vi "Acquire and Playback Data and Video LV2009.vi"() -> ()   [LabVIEW 2017]
uses:
  <vilib>/userdefined/High Color/IMAQdx.ctl
  <vilib>/DAQmx/read.llb/DAQmx Read (Analog Wfm 1Chan NSamp).vi
  <vilib>/DAQmx/create/channels.llb/DAQmx Create Channel (AI-Acceleration-Accelerometer).vi
  <vilib>/DAQmx/configure/timing.llb/DAQmx Timing (Sample Clock).vi
  <vilib>/DAQmx/miscellaneous.llb/DAQmx Fill In Error Info.vi
  <vilib>/vision/driver/NI_Vision_Acquisition_Software.lvlib
  <resource>/objmgr/daqmx.rc
panel:
  in  "Physical Channels":tag
  in  "AVI Path":path
  in  "Sampling Rate":dbl=1652.0
  in  "Stop Playback":bool
  in  "Tab Control":enum32{"Live Recording", "Playback"}(tab)
  out "Waveform Chart":waveform(dbl)(graph)={"t0"=timestamp(3330377079.0471377 s since 1904-01-01), "dt"=0.0005859375, "Y"=[0.0017552654709999996, 0.0017790570699999996, 0.0017997984639999997, 0.0018540921129999997, 0.0018882544089999997, 0.002001111994, 0.0019730501079999996, 0.0020255136339999997, 0.0021456917109999997, 0.0021944949909999995], "attributes"=variant("NI_ChannelName"=variant(string "cDAQ2Mod4/ai1"), "NI_UnitDescription"=variant(string "g"), "NI_dBReference"=variant(dbl 1.0))}
  out "Acquisition Video":T1(plugin-control)
  out "Waveform Chart 2":waveform(dbl)(graph)
  out "Playback Video":T1(plugin-control)
  out "Movie Progression":dbl(slide) max=500.0 scale=-1.0..335.0
  in  "Stop Acquisition":bool
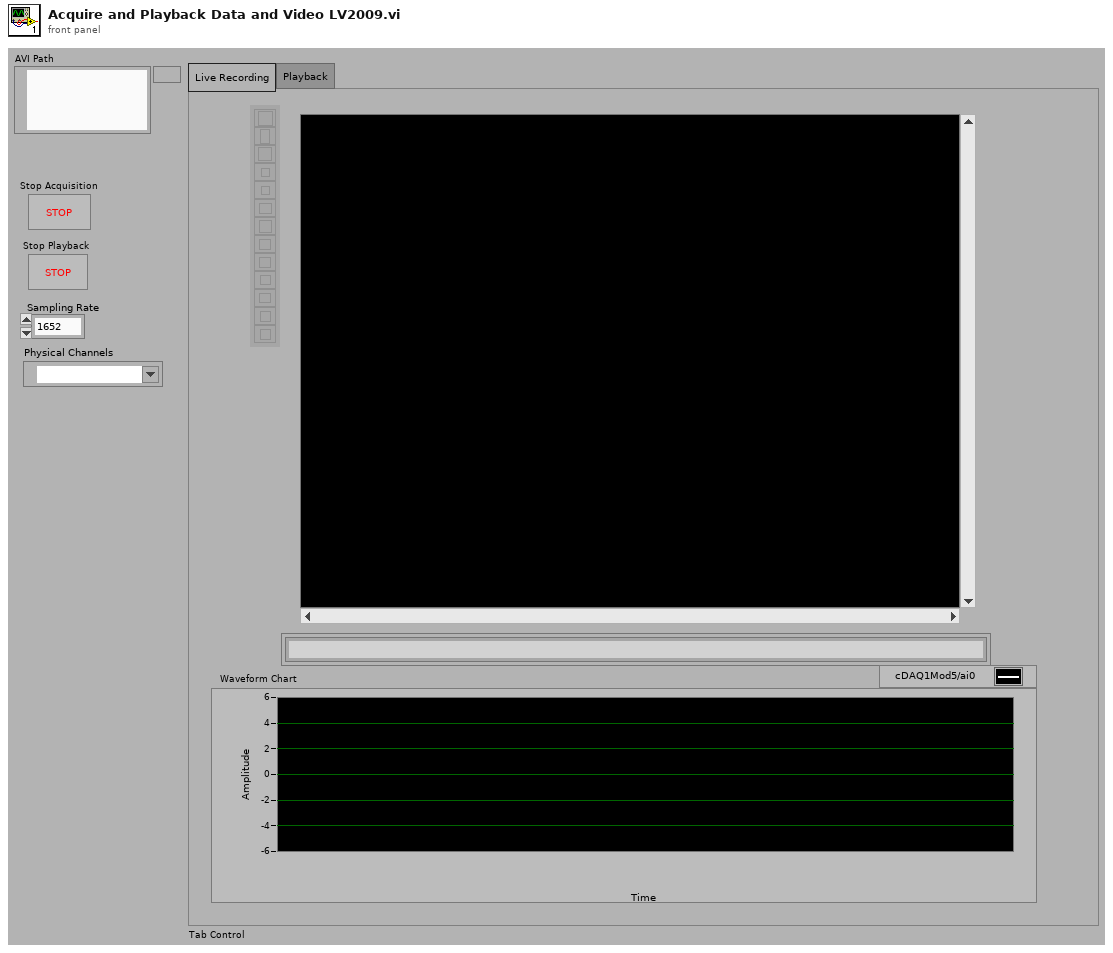
[diagram p1: front panel]
types:
  T1 = typedef "IMAQ Image.ctl" = refnum<image>
  T2 = typedef "IMAQdx.ctl" = refnum<k21>
  T3 = typedef "Image Type" = u32
  T4 = typedef "AviRefnum.ctl" = refnum<k1>
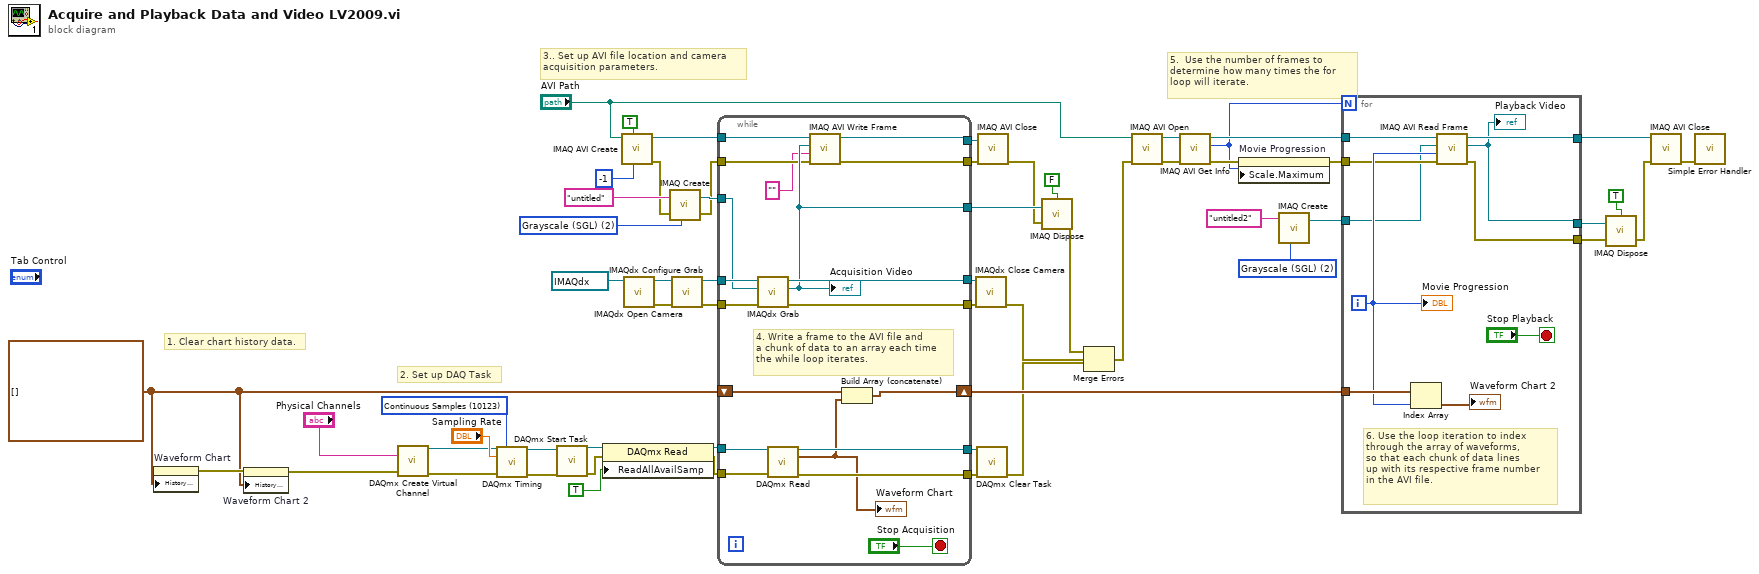
[diagram p0: block diagram]
diagram:
  w2 = waveform(dbl)[] [] ("History Data")
  w29 = T3 2 items=["Grayscale (U8)", "Grayscale (I16)", "Grayscale (SGL)", "Complex (CSG)", "RGB (U32)", "HSL (U32)", "RGB (U64)", "Grayscale (U16)"] ("Image Type")
  w35 = T3 2 items=["Grayscale (U8)", "Grayscale (I16)", "Grayscale (SGL)", "Complex (CSG)", "RGB (U32)", "HSL (U32)", "RGB (U64)", "Grayscale (U16)"] ("Image Type")
  w50 = 10123 items=["Finite Samples"=10178, "Continuous Samples"=10123, "Hardware Timed Single Point"=12522] ("sample mode")
  # "5.  Use the number of frames to \ndetermine how many times the for \nloop will iterate."
  # "3.. Set up AVI file location and camera \nacquisition parameters."
  # "2. Set up DAQ Task"
  # "1. Clear chart history data."
  n1 = property on="Waveform Chart" class="WFChart (strict)"("History Data"=w2) -> (error out=w4:errorcluster)  [unwired: 2 in, 1 out]
  n2 = property on="Waveform Chart 2" class="WFChart (strict)"(error in=w4, "History Data"=w2) -> (error out=w3:errorcluster)  [unwired: 1 in, 1 out]
  n3 = call-poly <vilib>:"DAQmx Create Virtual Channel.vi"("physical channels"="Physical Channels", "error in"=w3) -> ("task out"=w37:refnum<k21>, "error out"=w48:errorcluster)  [unwired: 11 in, 1 out]
  n4 = call-poly <vilib>:"DAQmx Timing.vi"("task/channels in"=w37, "sample mode"=w50, "rate"="Sampling Rate", "error in"=w48) -> ("task out"=w47:refnum<k21>, "error out"=w46:errorcluster)  [unwired: 3 in, 7 out]
  n5 = call <vilib>:"DAQmx Start Task.vi"("task/channels in"=w47, "error in"=w46) -> ("task out"=w12:refnum<k21>, "error out"=w13:errorcluster)  [unwired: 12 out]
  n6 = property class="DAQmx Read"(reference=w12, error in=w13, "ReadAllAvailSamp"=TRUE) -> (reference out=w11:refnum<k21>, error out=w10:errorcluster)
  n7 = call "IMAQ AVI Create"("quality"=-1, "Has Data"=TRUE, "AVI Path"="AVI Path") -> ("error out"=w39:errorcluster, "Avi Refnum"=w52:T4)  [unwired: 4 in, 3 out]
  n8 = call <vilib>:"IMAQdx Open Camera.vi"("Session In"=T2 "cam4") -> ("error out"=w42:errorcluster, "Session Out"=w43:T2)  [unwired: 2 in, 7 out]
  n9 = call "IMAQ Create"("Image Name"="untitled", "Image Type"=w35, "error in (no error)"=w39) -> ("New Image"=w56:T1, "error out"=w51:errorcluster)  [unwired: 1 in, 1 out]
  n10 = call <vilib>:"IMAQdx Configure Grab.vi"("error in"=w42, "Session In"=w43) -> ("error out"=w57:errorcluster, "Session Out"=w58:T2)  [unwired: 8 out]
  n11 = while {
    tunnel: w58 -> [w77]
    tunnel: w57 -> [w76]
    tunnel: w56 -> [w75]
    tunnel: [w74] -> w55
    tunnel: [w73] -> w54
    tunnel: [w72] -> w53
    tunnel: w52 -> [w71]
    tunnel: w51 -> [w70]
    tunnel: w11 -> [w69]
    tunnel: w10 -> [w68]
    tunnel: [w67] -> w45
    tunnel: [w66] -> w44
    tunnel: [w65] -> w23
    tunnel: [w64] -> w19
    shift-right: [w61] -> w9
    shift-left: w2 -> [w62]
    stop <- "Stop Acquisition" stop-if-true
    # "4. Write a frame to the AVI file and \na chunk of data to an array each time\nthe while loop iterates."
    n12 = call <vilib>:"IMAQdx Grab.vi"("error in"=w76, "Image In"=w75, "Session In"=w77) -> ("error out"=w73:errorcluster, "Image Out"=w72:T1, "Session Out"=w74:T2)  [unwired: 1 in, 5 out]
    "Acquisition Video" <- w72
    n13 = call-poly <vilib>:"DAQmx Read.vi"("task/channels in"=w69, "error in"=w68) -> ("task out"=w67:refnum<k21>, "data"=w60:waveform(dbl), "error out"=w66:errorcluster)  [unwired: 1 in, 10 out]
    "Waveform Chart" <- w60
    n14 = call "IMAQ AVI Write Frame"("error in (no error)"=w70, "Data"="", "Image"=w72, "Avi Refnum"=w71) -> ("error out"=w64:errorcluster, "Avi Refnum (duplicate)"=w65:T4)  [unwired: 6 out]
    n15 = Build Array (concatenate)(w62, w60) -> (w61:waveform(dbl)[])
  }
  n16 = call <vilib>:"IMAQdx Close Camera.vi"("error in"=w54, "Session In"=w55) -> ("error out"=w6:errorcluster)  [unwired: 9 out]
  n17 = call <vilib>:"DAQmx Clear Task.vi"("task in"=w45, "error in"=w44) -> ("error out"=w5:errorcluster)  [unwired: 13 out]
  n18 = call "IMAQ AVI Close"("error in (no error)"=w19, "Avi Refnum"=w23) -> ("error out"=w18:errorcluster)  [unwired: 9 out]
  n19 = call "IMAQ Dispose"("All Images? (No)"=FALSE, "Image"=w53, "error in (no error)"=w18) -> ("error out"=w7:errorcluster)  [unwired: 3 out]
  n20 = Merge Errors(w7, w6, w5) -> (w8:errorcluster)
  n21 = call "IMAQ AVI Open"("error in (no error)"=w8, "AVI Path"="AVI Path") -> ("error out"=w21:errorcluster, "Avi Refnum"=w22:T4)  [unwired: 8 out]
  n22 = call "IMAQ AVI Get Info"("error in (no error)"=w21, "Avi Refnum"=w22) -> ("error out"=w28:errorcluster, "Number of Frames"=w17:u32, "Avi Refnum (duplicate)"=w27:T4)  [unwired: 7 out]
  n23 = property on="Movie Progression" class="Slide (strict)"(error in=w28, "Scale.Maximum"=w17) -> (error out=w1:errorcluster)  [unwired: 1 in, 1 out]
  n24 = call "IMAQ Create"("Image Name"="untitled2", "Image Type"=w29) -> ("New Image"=w25:T1)  [unwired: 2 in, 2 out]
  n25 = for {
    N: w17 -> [_]
    tunnel: [w87] -> w34
    tunnel: [w86] -> w31
    tunnel: w27 -> [w85]
    tunnel: [w78] -> w26
    tunnel: w25 -> [w79]
    tunnel: w9 -> [w84]
    tunnel: w1 -> [w80]
    i -> [w82]
    stop <- "Stop Playback" stop-if-true
    # "6. Use the loop iteration to index\nthrough the array of waveforms, \nso that each chunk of data lines\nup with its respective frame number\nin the AVI file."
    n26 = Index Array(array=w84, index=w82) -> (element=→"Waveform Chart 2":waveform(dbl))
    n27 = call "IMAQ AVI Read Frame"("error in (no error)"=w80, "Frame Number"=w82, "Image"=w79, "Avi Refnum"=w85) -> ("error out"=w86:errorcluster, "Image Out"=w78:T1, "Avi Refnum (duplicate)"=w87:T4)  [unwired: 1 in, 4 out]
    "Playback Video" <- w78
    "Movie Progression" <- w82
  }
  n28 = call "IMAQ Dispose"("All Images? (No)"=TRUE, "Image"=w26, "error in (no error)"=w31) -> ("error out"=w30:errorcluster)  [unwired: 3 out]
  n29 = call "IMAQ AVI Close"("error in (no error)"=w30, "Avi Refnum"=w34) -> ("error out"=w33:errorcluster)  [unwired: 9 out]
  n30 = call <vilib>:"Simple Error Handler.vi"("error in (no error)"=w33) -> ()  [unwired: 1 in, 8 out]
